vi "Initialize_IMU.vi"(10 "orientation":u32(ring)=136 items=["ORIENTATION_Z_UP"=136, "ORIENTATION_Z_DOWN"=396, "ORIENTATION_X_UP"=14, "ORIENTATION_X_DOWN"=266, "ORIENTATION_Y_UP"=112, "ORIENTATION_Y_DOWN"=336], 11 "enable_magnetometer":i32) -> (0 "error out":errorcluster, 2 "gyro_fsr":u32(ring)=2 items=["G_FSR_250DPS"=250, "G_FSR_500DPS"=500, "G_FSR_1000DPS"=1000, "G_FSR_2000DPS"=2000], 3 "data out":T1)   [LabVIEW 2014]
uses:
  <userlib>/UCSD Robotics Lab/Robotics-Cape/LV/libroboticscape.lvlib
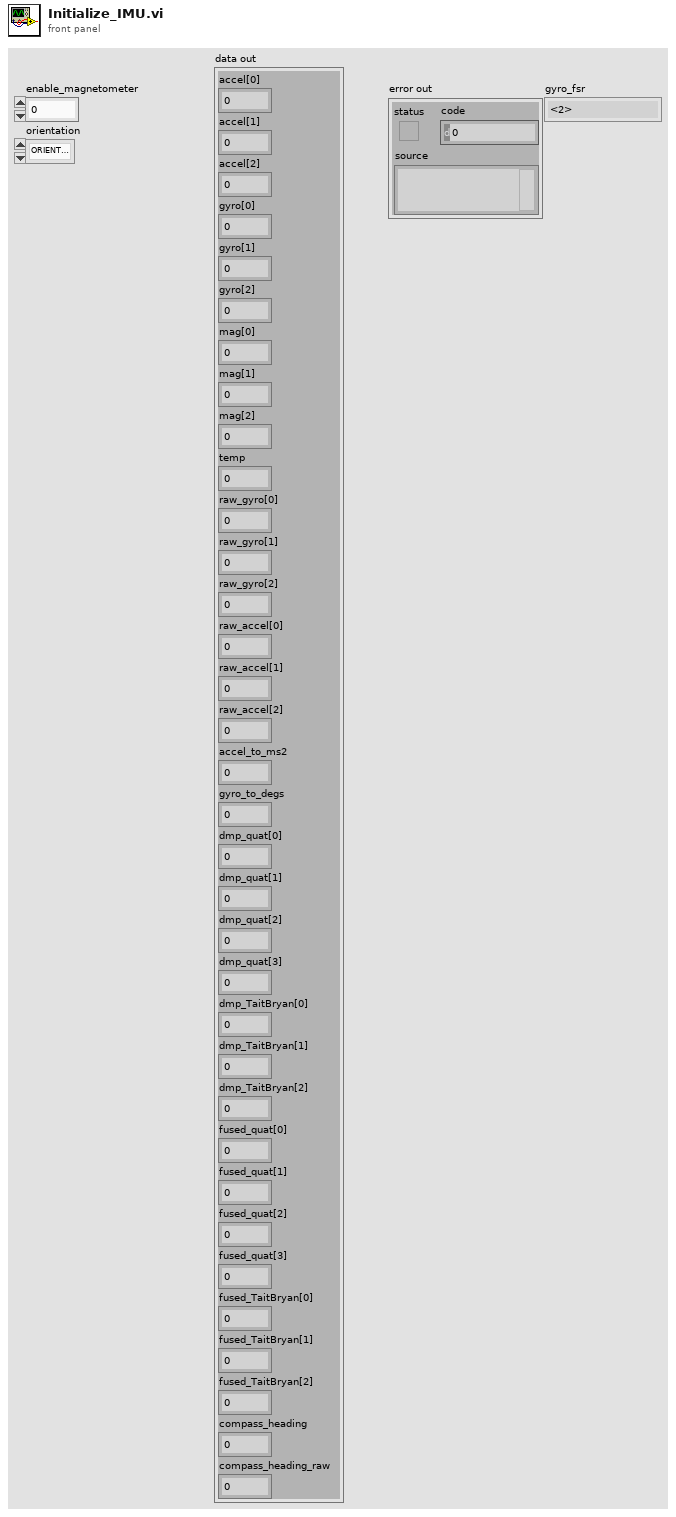
[diagram p1: front panel]
types:
  T1 = cluster{"accel[0]":sgl, "accel[1]":sgl, "accel[2]":sgl, "gyro[0]":sgl, "gyro[1]":sgl, "gyro[2]":sgl, "mag[0]":sgl, "mag[1]":sgl, "mag[2]":sgl, "temp":sgl, "raw_gyro[0]":i16, "raw_gyro[1]":i16, "raw_gyro[2]":i16, "raw_accel[0]":i16, "raw_accel[1]":i16, "raw_accel[2]":i16, "accel_to_ms2":sgl, "gyro_to_degs":sgl, "dmp_quat[0]":sgl, "dmp_quat[1]":sgl, "dmp_quat[2]":sgl, "dmp_quat[3]":sgl, "dmp_TaitBryan[0]":sgl, "dmp_TaitBryan[1]":sgl, "dmp_TaitBryan[2]":sgl, "fused_quat[0]":sgl, "fused_quat[1]":sgl, "fused_quat[2]":sgl, "fused_quat[3]":sgl, "fused_TaitBryan[0]":sgl, "fused_TaitBryan[1]":sgl, "fused_TaitBryan[2]":sgl, "compass_heading":sgl, "compass_heading_raw":sgl}
  T2 = cluster{"accel_fsr":u32, "gyro_fsr":u32, "gyro_dlpf":u32, "accel_dlpf":u32, "enable_magnetometer":i32, "dmp_sample_rate":i32, "orientation":u32, "compass_mix_factor":i32, "dmp_interrupt_priority":i32, "show_warnings":i32}
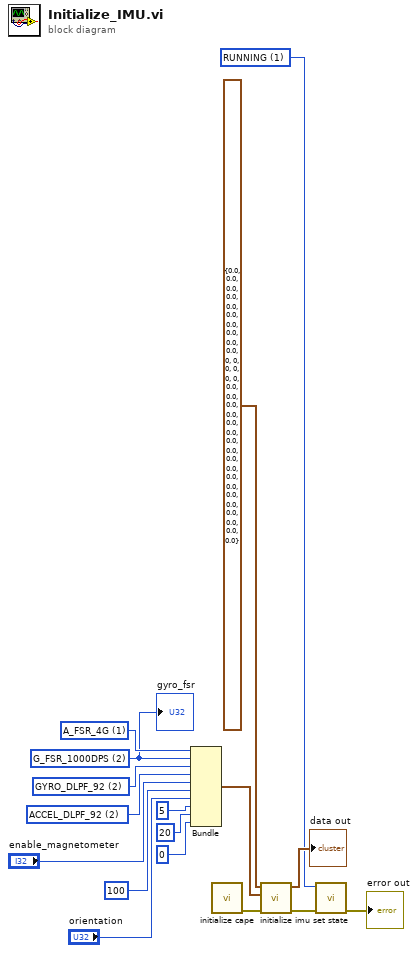
[diagram p0: block diagram]
diagram:
  w11 = u32 1 items=["A_FSR_2G", "A_FSR_4G", "A_FSR_8G", "A_FSR_16G"] ("accel_fsr")
  w10 = u32 2 items=["G_FSR_250DPS", "G_FSR_500DPS", "G_FSR_1000DPS", "G_FSR_2000DPS"] ("gyro_fsr")
  w9 = u32 2 items=["GYRO_DLPF_OFF", "GYRO_DLPF_184", "GYRO_DLPF_92", "GYRO_DLPF_41", "GYRO_DLPF_20", "GYRO_DLPF_10", "GYRO_DLPF_5"] ("gyro_dlpf")
  w8 = u32 2 items=["ACCEL_DLPF_OFF", "ACCEL_DLPF_184", "ACCEL_DLPF_92", "ACCEL_DLPF_41", "ACCEL_DLPF_20", "ACCEL_DLPF_10", "ACCEL_DLPF_5"] ("accel_dlpf")
  w13 = u32 1 items=["UNINITIALIZED", "RUNNING", "PAUSED", "EXITING"] ("new_state")
  n1 = Bundle("accel_fsr"=w11, "gyro_fsr"=w10, "gyro_dlpf"=w9, "accel_dlpf"=w8, "enable_magnetometer"="enable_magnetometer", "dmp_sample_rate"=100, "orientation"="orientation", "compass_mix_factor"=5, "dmp_interrupt_priority"=20, "show_warnings"=0) -> (w1:T2)  [unwired: 1 in]
  n2 = call <userlib>:"initialize cape.vi"() -> ("error out"=w15:errorcluster)  [unwired: 10 in, 1 out]
  n3 = call <userlib>:"initialize imu.vi"("error in (no error)"=w15, "Cluster"=w1, "data"=T1 {"accel[0]"=0.0, "accel[1]"=0.0, "accel[2]"=0.0, "gyro[0]"=0.0, "gyro[1]"=0.0, "gyro[2]"=0.0, "mag[0]"=0.0, "mag[1]"=0.0, "mag[2]"=0.0, "temp"=0.0, "raw_gyro[0]"=0, "raw_gyro[1]"=0, "raw_gyro[2]"=0, "raw_accel[0]"=0, "raw_accel[1]"=0, "raw_accel[2]"=0, "accel_to_ms2"=0.0, "gyro_to_degs"=0.0, "dmp_quat[0]"=0.0, "dmp_quat[1]"=0.0, "dmp_quat[2]"=0.0, "dmp_quat[3]"=0.0, "dmp_TaitBryan[0]"=0.0, "dmp_TaitBryan[1]"=0.0, "dmp_TaitBryan[2]"=0.0, "fused_quat[0]"=0.0, "fused_quat[1]"=0.0, "fused_quat[2]"=0.0, "fused_quat[3]"=0.0, "fused_TaitBryan[0]"=0.0, "fused_TaitBryan[1]"=0.0, "fused_TaitBryan[2]"=0.0, "compass_heading"=0.0, "compass_heading_raw"=0.0}) -> ("error out"=w14:errorcluster, "data out"=→"data out":T1)  [unwired: 4 in, 1 out]
  n4 = call <userlib>:"set state.vi"("error in (no error)"=w14, "new_state"=w13) -> ("error out"=→"error out":errorcluster)  [unwired: 8 in, 1 out]
  "gyro_fsr" <- w10
